vi "ParseMsg.vi"(8 "error in (no error)":errorcluster, 10 "ToParse":string, 11 "Popup Msg in":refnum<class "Popup Msg.lvclass">) -> (0 "error out":errorcluster, 3 "Popup Msg out":refnum<class "Popup Msg.lvclass">)   [LabVIEW 2020, in "Test-Client.lvlib" / "Popup Msg.lvclass"]
uses:
  Popup Msg.lvclass
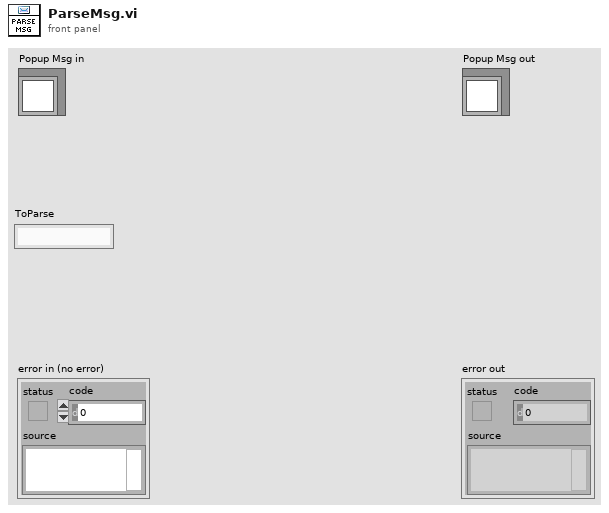
[diagram p1: front panel]
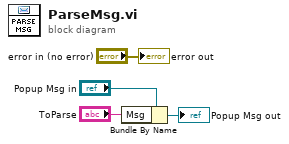
[diagram p0: block diagram]
diagram:
  n1 = Bundle By Name(cluster="Popup Msg in", "Msg"="ToParse") -> (→"Popup Msg out":refnum<class "Popup Msg.lvclass">)
  "error out" <- "error in (no error)"
